vi "Translation_Create.vi"(10 "Y":dbl, 11 "X":dbl) -> (3 "TRANSLATION":T1)   [LabVIEW 2019, in "PathExecution_Library.lvlib"]
uses:
  PathExecution_Library.lvlib
  TRANSLATION.ctl
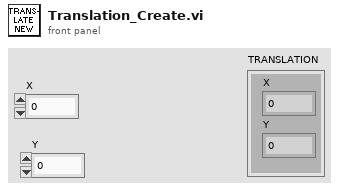
[diagram p1: front panel]
types:
  T1 = typedef "PathExecution_Library.lvlib/TRANSLATION.ctl" = cluster{"X":dbl, "Y":dbl}
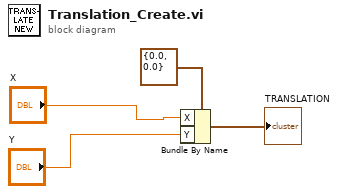
[diagram p0: block diagram]
diagram:
  n1 = Bundle By Name(cluster=T1 {"X"=0.0, "Y"=0.0} ("TRANSLATION"), "X"="X", "Y"="Y") -> (→"TRANSLATION":T1)
